vi "set_LaserFireThreshold.vi"() -> ()   [LabVIEW 2014]
panel:
  in  "Num Bytes to Fetch (64)":u8=64 min=1
  out "error out":errorcluster
  in  "error in (no error)":errorcluster
  in  "Address (0x50)":u16=80 max=1023 format="%.0x"
  in  "Aardvark Handle":i32 min=0
  in  "Threshold":dbl
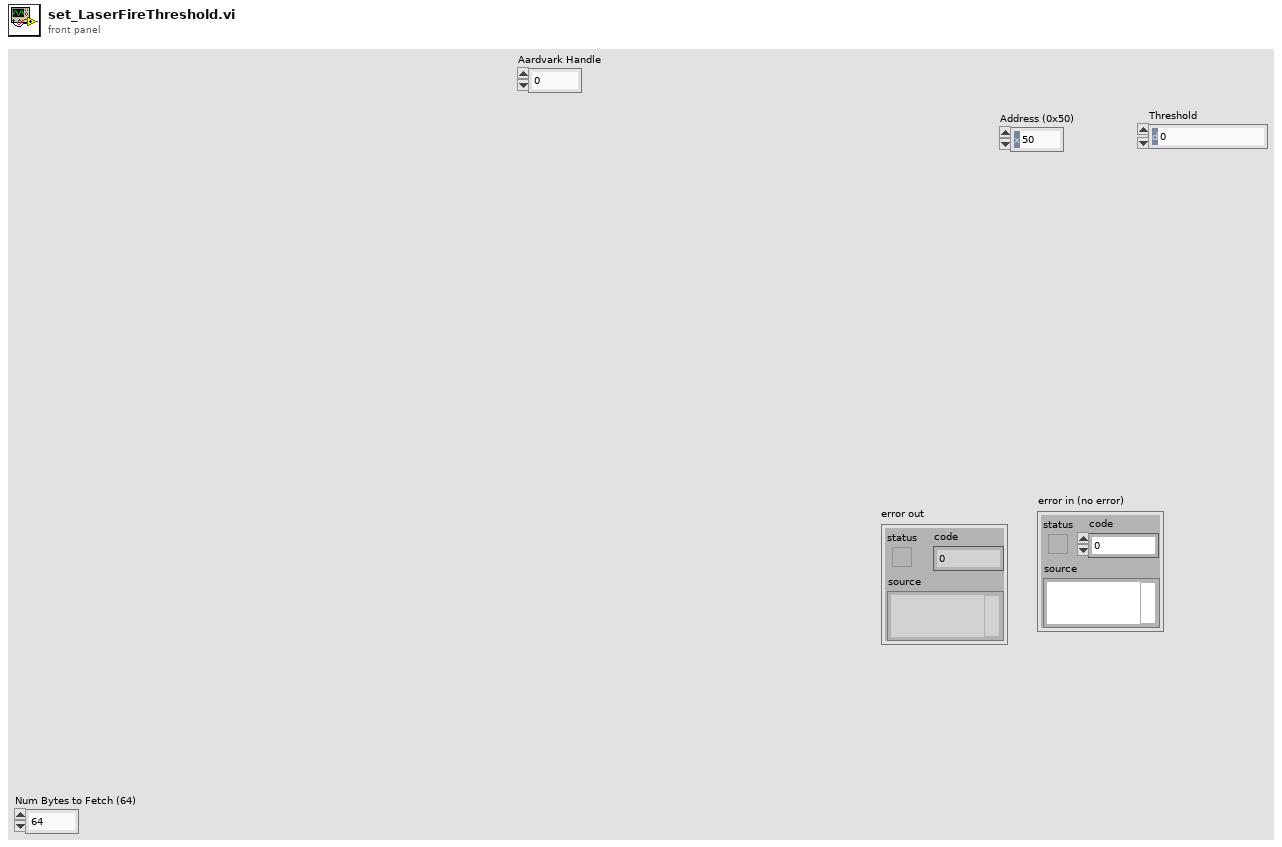
[diagram p1: front panel]
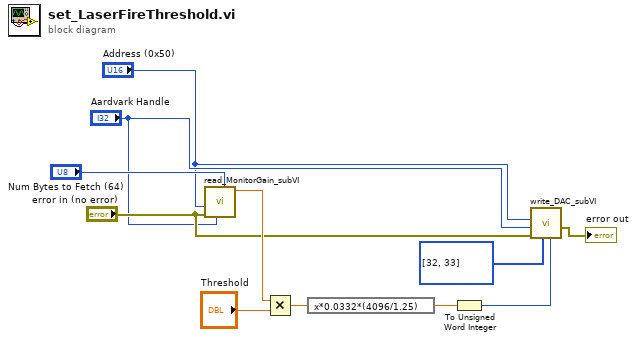
[diagram p0: block diagram]
diagram:
  n1 = call "read_MonitorGain_subVI.vi"("Num Bytes to Fetch (64) in"="Num Bytes to Fetch (64)", "Aardvark Handle in"="Aardvark Handle", "error in (no error)"="error in (no error)", "Address (0x50) in"="Address (0x50)") -> ("Gain"=w7:dbl)  [unwired: 7 in]
  n2 = Multiply(x=w7, y="Threshold") -> (x*y=w9:dbl)
  n3 = expression code="x*0.0332*(4096/1.25)"(w9) -> (w11:dbl)
  n4 = To Unsigned Word Integer(number=w11) -> (unsigned 16bit integer=w2:u16)
  n5 = call "write_DAC_subVI.vi"("DAC_Val"=w2, "DAC_ADD"=u8[] [32, 33], "error in (no error)"="error in (no error)", "Aardvark Handle in"="Aardvark Handle", "Address (0x50) in"="Address (0x50)") -> ("error out"=→"error out":errorcluster)  [unwired: 6 in]
